vi "FormMain.vi"() -> ()   [LabVIEW 2012]
uses:
  S7Ref.vi
  resultShow.vi
panel:
  out "涂线束色标":bool
  out "请安装线束":bool
  in  "管柱码":string
  in  "countLeft":u32
  out "拾取下轴固定螺丝":bool
  out "安装下轴左转两圈检测":bool=TRUE
  in  "判定设定 2":string[][](table)
  in  "参数设定 2":string[][](table)
  out "takesTime":string
  out "表格控件":string[][](table)
  out "FFT范围 2":string[][](table)
  out "翻起下轴后按左启动按钮下轴平台复位":bool
  out "外泄漏":bool
  out "自由间隙":bool
  out "右转两圈检测":bool
  out "请给总成扫码":bool=TRUE
  out "涂下轴色标":bool
  out "输出扭矩":dbl caption="数值 24" format="%.1f Nm"
  in  "打开按钮":bool
  in  "自动":bool
  out "rigStatus":string="提示信息"
  out "connectionMode":string
  out "productsName":string
  out "userStatus":string
  out "userName":string
  out "双手按启动按钮夹紧工件顶升下轴平台":bool
  out "一号气枪安装下轴":bool=TRUE
  out "双手启动翻转":bool
  out "主观判断是否合格":bool
  out "拆卸下轴后双手启动翻转平位":bool
  out "按右启动键取出工件":bool
  # "下轴总成装配及主观异响鉴别"
  # "广东和氏自动化技术股份有限公司"
  # "GUANGDONG HESH AUTOMATION TECHNOLOGY CO.,LTD."
  # "安装步骤"
  # "完成计数："
  # "："
  # "用时："
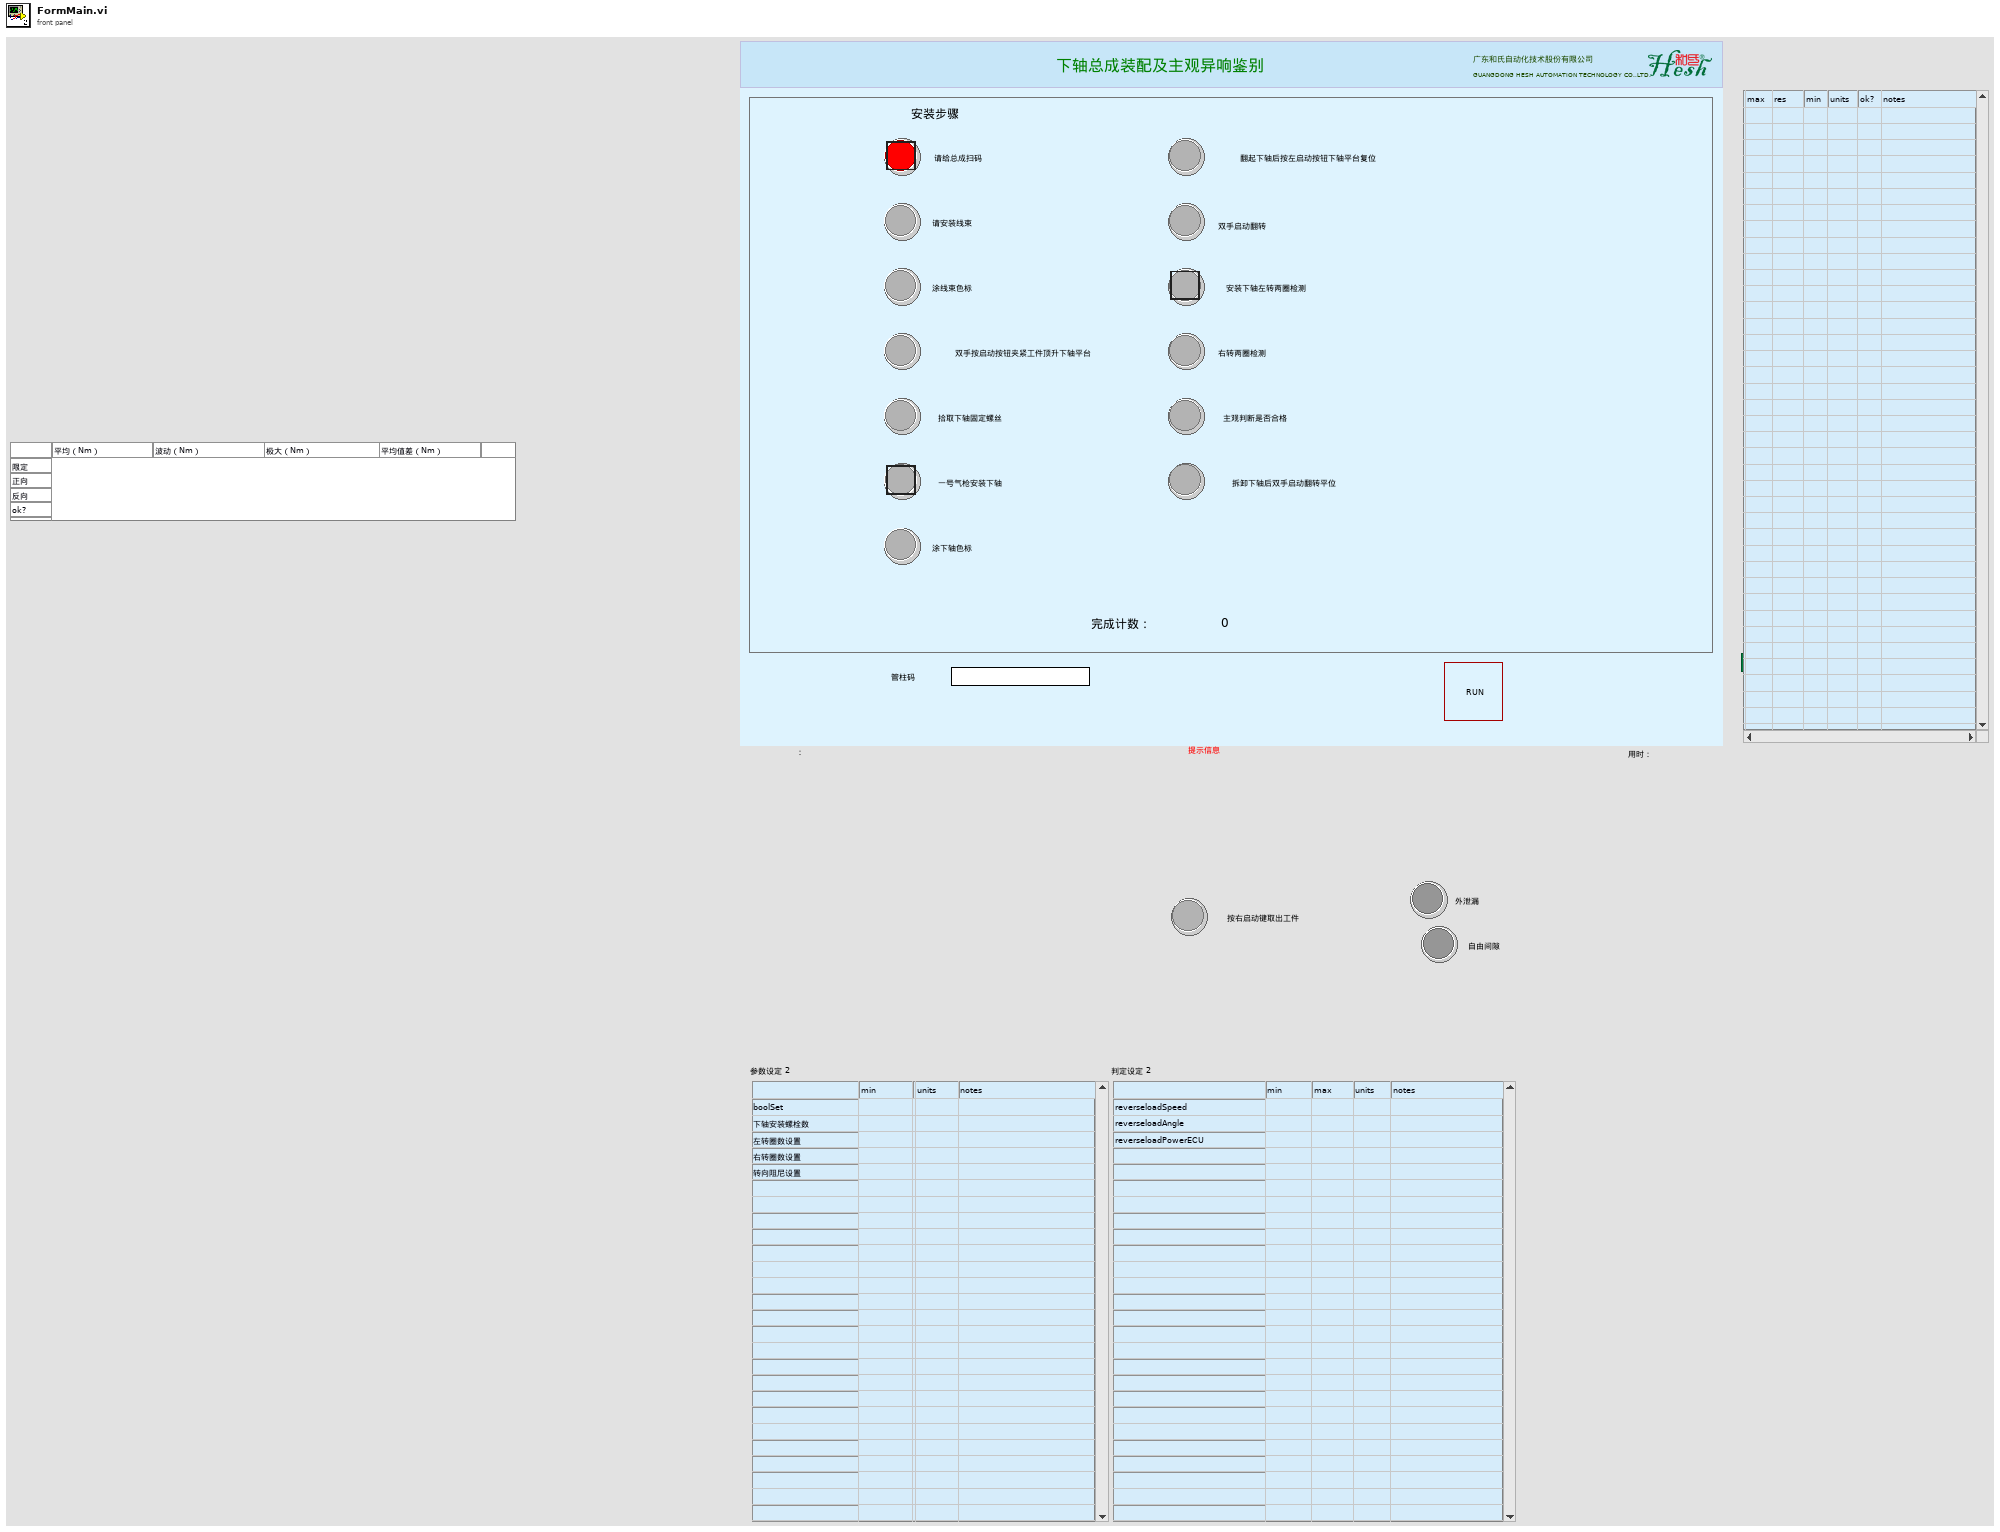
[diagram p1: front panel]
types:
  T1 = enum32{"Invalid", "Standard", "Closed", "Hidden", "Minimized", "Maximized"}
  T2 = cluster{"takesTime":refnum<vi>, "userStatus":refnum<vi>, "userName":refnum<vi>, "connectionMode":refnum<vi>, "productsName":refnum<vi>, "rigStatus":refnum<vi>, "管柱码":refnum<vi>}
  T3 = cluster{"userCode":string, "userName":string, "userStatus":string, "connectionMode":string, "takesTime":string, "countDone":string, "countOK":string, "countNG":string, "rigStatus":string, "productsName":string, "partCode1":string, "partCode2":string, "partCode3":string}
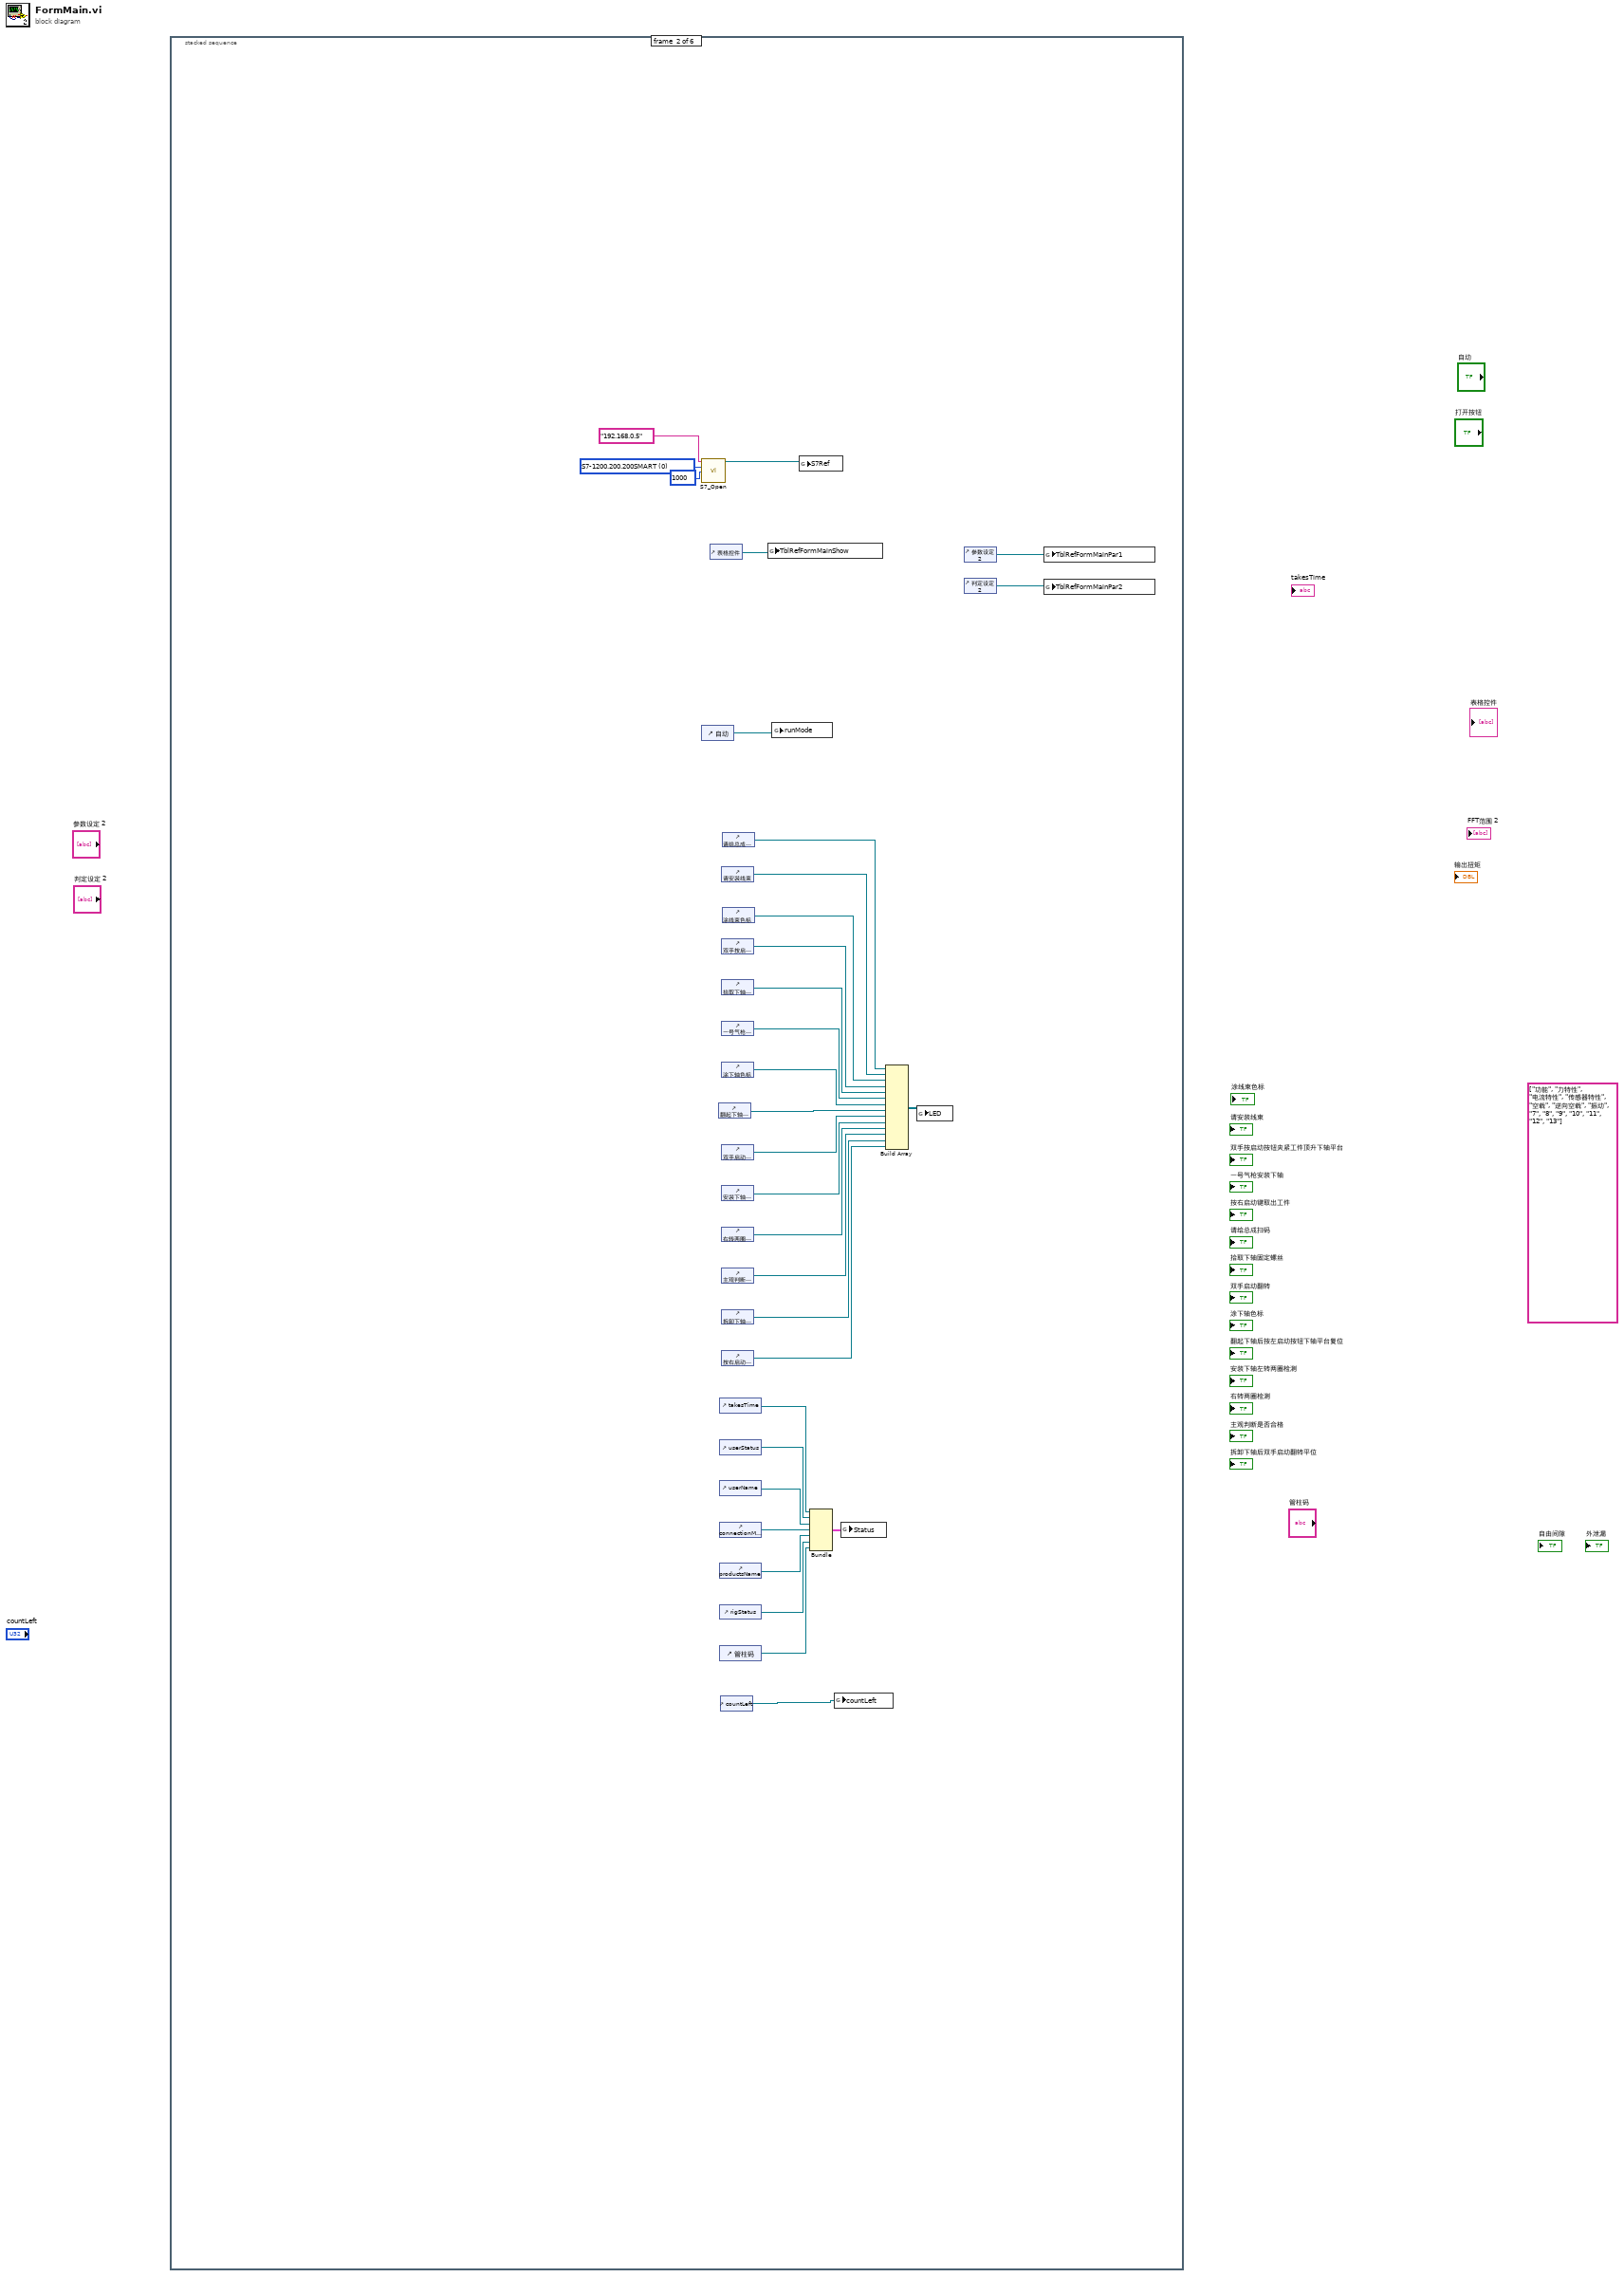
[diagram p0: block diagram]
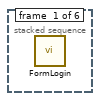
[diagram p2: hidden frame]
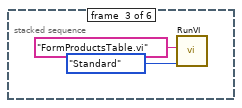
[diagram p3: hidden frame]
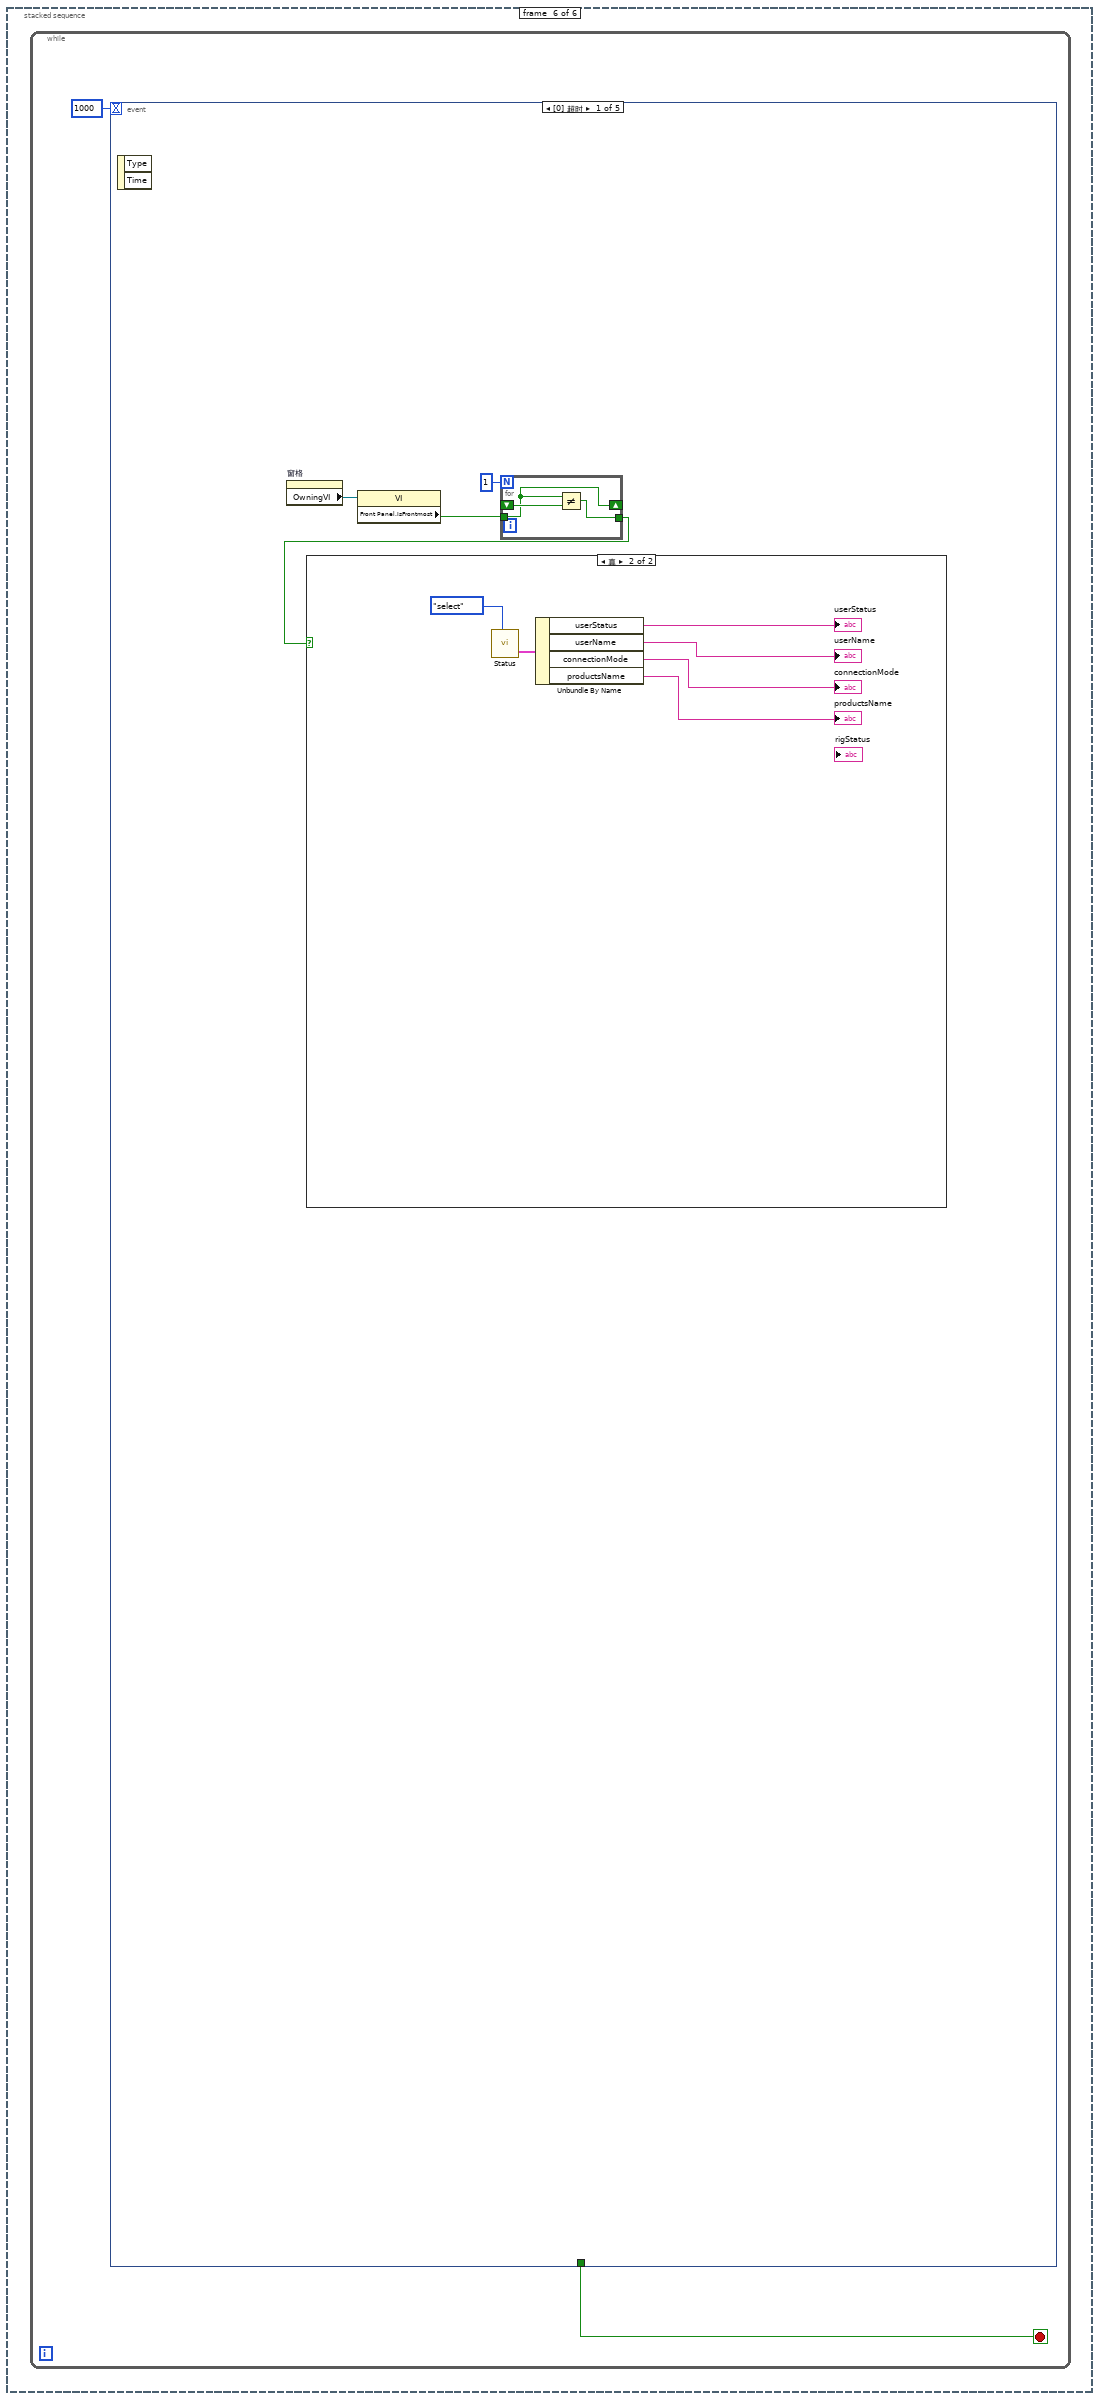
[diagram p6: hidden frame]
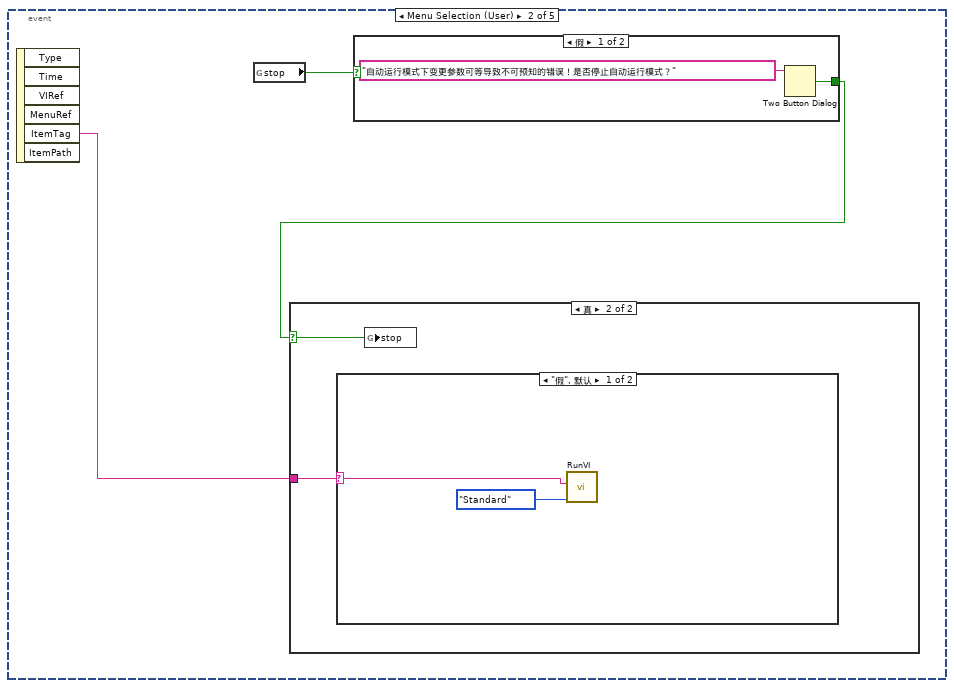
[diagram p8: hidden frame]
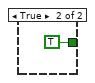
[diagram p9: hidden frame]
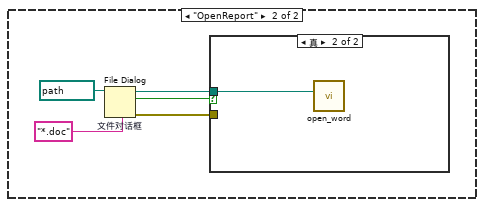
[diagram p11: hidden frame]
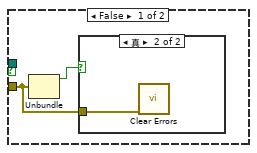
[diagram p12: hidden frame]
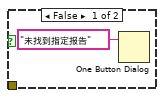
[diagram p13: hidden frame]
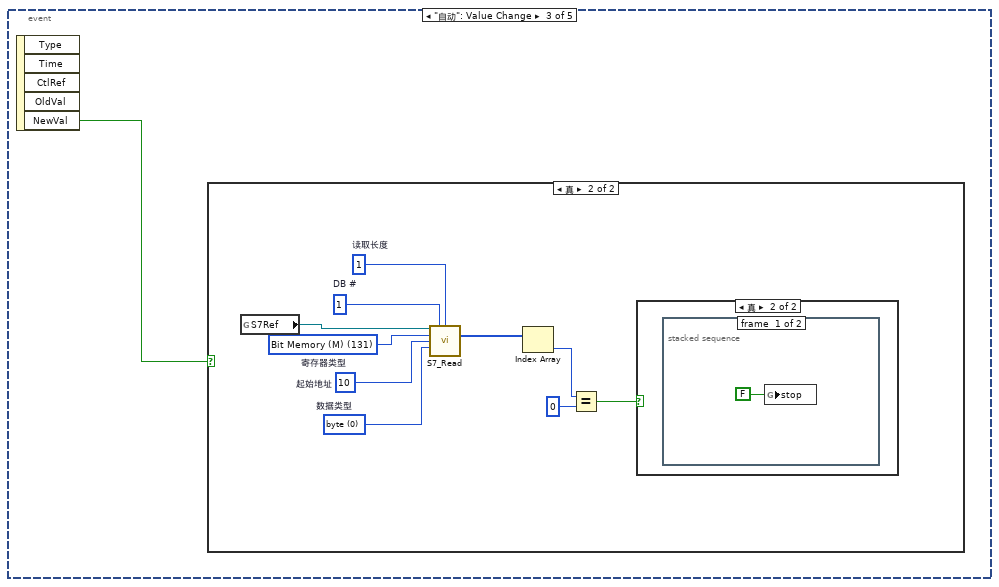
[diagram p14: hidden frame]
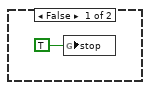
[diagram p15: hidden frame]
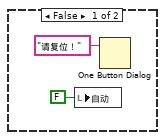
[diagram p16: hidden frame]
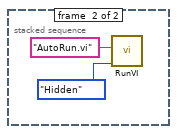
[diagram p17: hidden frame]
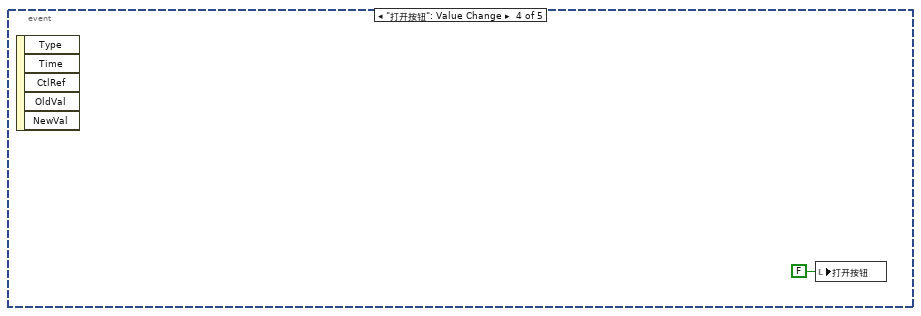
[diagram p18: hidden frame]
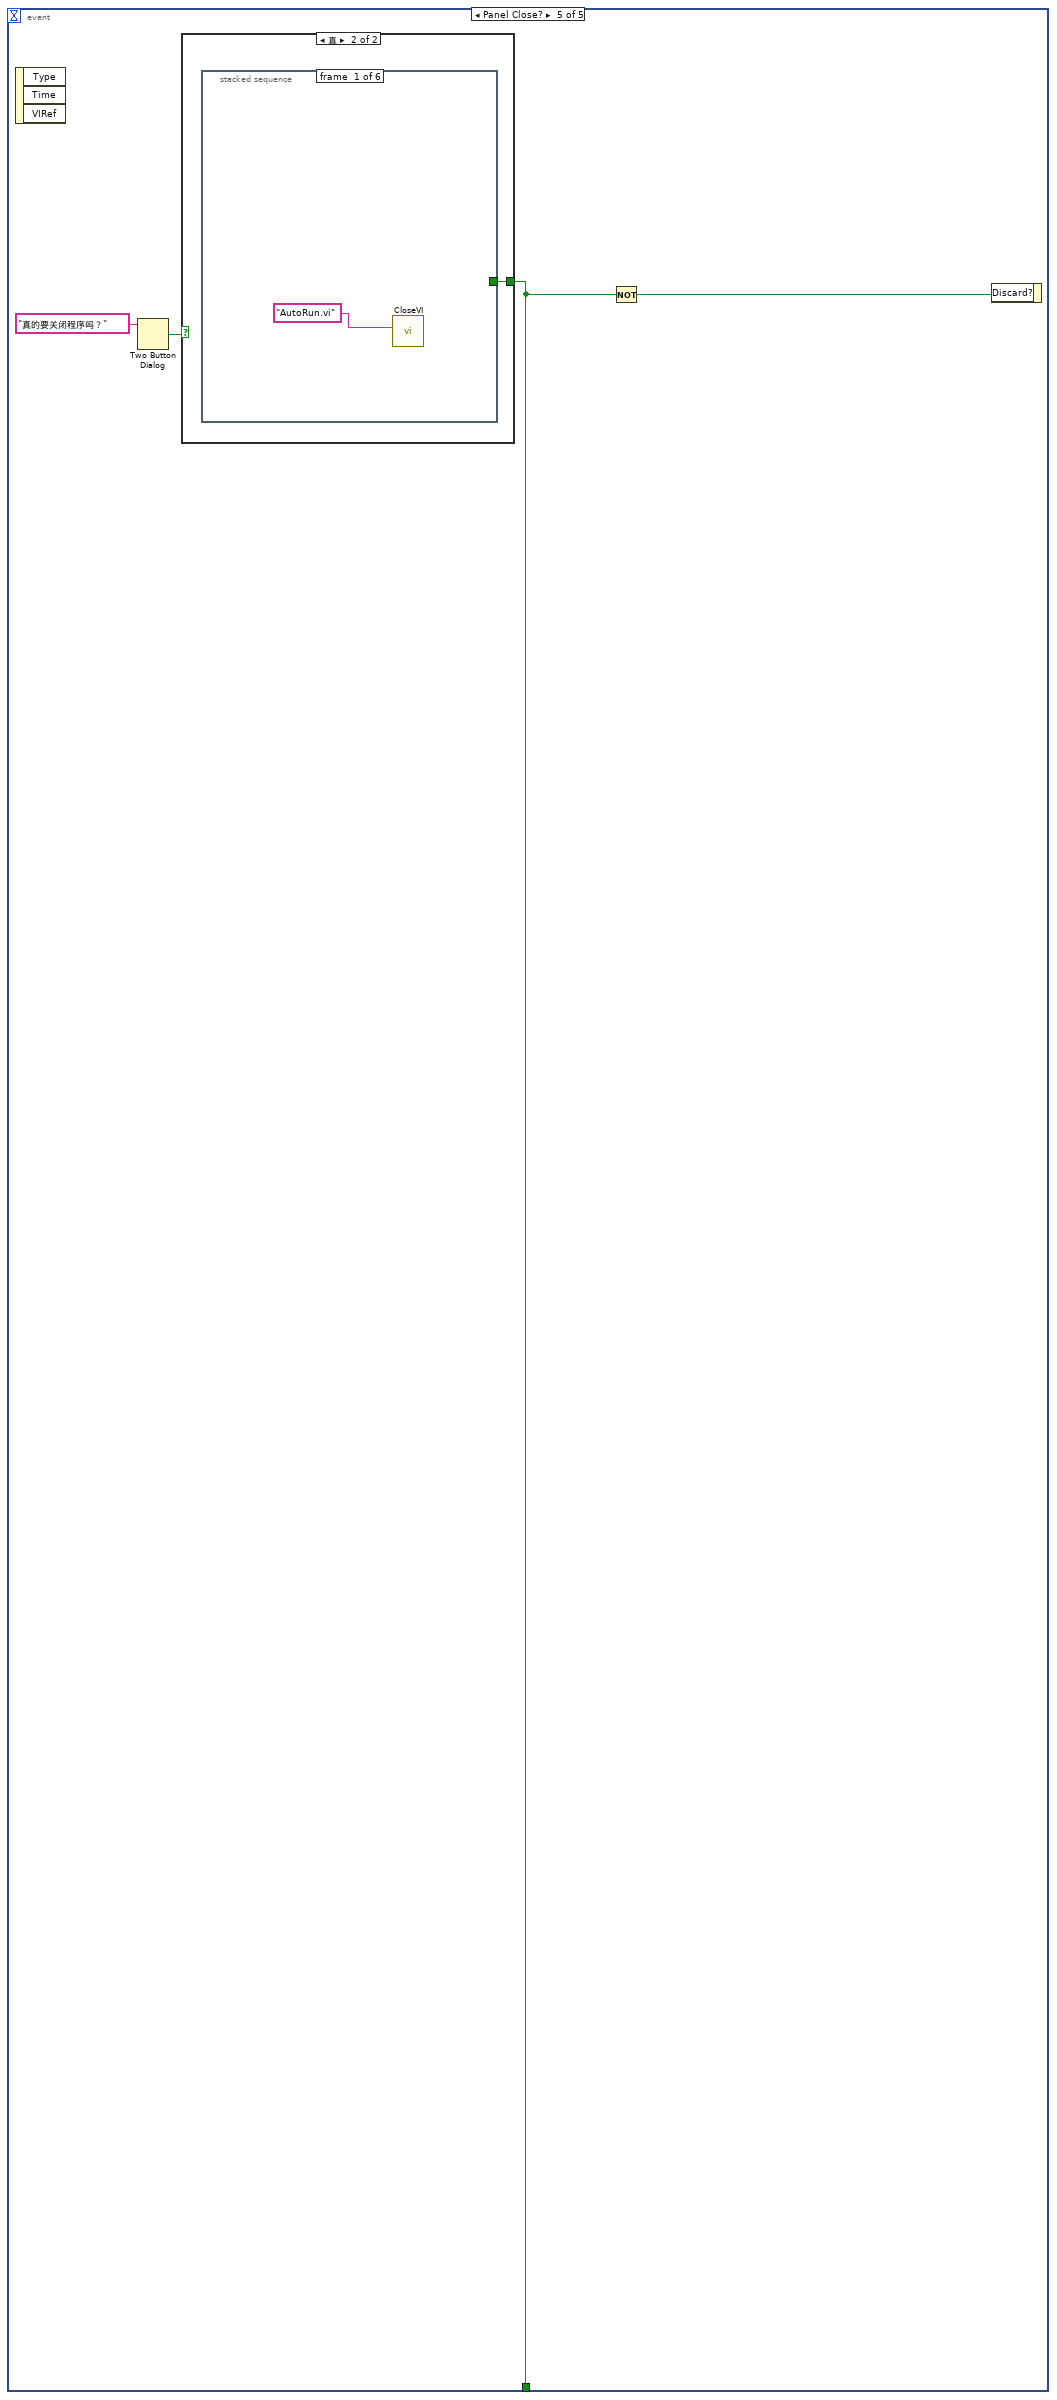
[diagram p19: hidden frame]
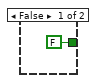
[diagram p20: hidden frame]
diagram:
  (unwired) string[] ["功能", "力特性", "电流特性", "传感器特性", "空载", "逆向空载", "振动", "7", "8", "9", "10", "11", "12", "13"] ("字符串[]")
  n1 = stacked-sequence {
    frame #0 {
      n2 = call "FormLogin.vi"() -> ()  [unwired: 12 in]
    }
    frame #1 {
      w30 = u8 0 items=["S7-1200.200.200SMART"=0, "S7-300"=2, "S7-400"=3] ("PLC 系列")
      n3 = call "S7_Open.vi"("IP 地址"="192.168.0.5", "PLC 系列"=w30, "超时（MS）"=1000) -> ("TCP"=w28:refnum<k5>)  [unwired: 10 in, 2 out]
      n4 = control-ref of="自动"() -> (w27:refnum<vi>)
      n5 = control-ref of="表格控件"() -> (w32:refnum<vi>)
      n6 = control-ref of="翻起下轴后按左启动按钮下轴平台复位"() -> (w4:refnum<vi>)
      n7 = control-ref of="takesTime"() -> (w15:refnum<vi>)
      n8 = control-ref of="userStatus"() -> (w21:refnum<vi>)
      n9 = control-ref of="userName"() -> (w20:refnum<vi>)
      n10 = control-ref of="connectionMode"() -> (w19:refnum<vi>)
      n11 = control-ref of="productsName"() -> (w18:refnum<vi>)
      n12 = control-ref of="rigStatus"() -> (w17:refnum<vi>)
      n13 = control-ref of="管柱码"() -> (w5:refnum<vi>)
      n14 = control-ref of="countLeft"() -> (w12:refnum<vi>)
      n15 = control-ref of="请安装线束"() -> (w2:refnum<vi>)
      n16 = control-ref of="双手按启动按钮夹紧工件顶升下轴平台"() -> (w10:refnum<vi>)
      n17 = control-ref of="拾取下轴固定螺丝"() -> (w8:refnum<vi>)
      n18 = control-ref of="一号气枪安装下轴"() -> (w22:refnum<vi>)
      n19 = control-ref of="涂下轴色标"() -> (w9:refnum<vi>)
      n20 = control-ref of="双手启动翻转"() -> (w23:refnum<vi>)
      n21 = control-ref of="安装下轴左转两圈检测"() -> (w7:refnum<vi>)
      n22 = control-ref of="右转两圈检测"() -> (w6:refnum<vi>)
      n23 = control-ref of="主观判断是否合格"() -> (w24:refnum<vi>)
      n24 = control-ref of="拆卸下轴后双手启动翻转平位"() -> (w25:refnum<vi>)
      n25 = control-ref of="按右启动键取出工件"() -> (w26:refnum<vi>)
      n26 = control-ref of="请给总成扫码"() -> (w3:refnum<vi>)
      n27 = control-ref of="涂线束色标"() -> (w1:refnum<vi>)
      n28 = global write "resultShow.vi" "TblRefFormMainShow"(w32) -> ()
      n29 = global write "resultShow.vi" "runMode"(w27) -> ()
      n30 = global write "S7Ref.vi" "S7Ref"(w28) -> ()
      n31 = Bundle("takesTime"=w15, "userStatus"=w21, "userName"=w20, "connectionMode"=w19, "productsName"=w18, "rigStatus"=w17, "管柱码"=w5) -> (w16:T2)  [unwired: 1 in]
      n32 = global write "resultShow.vi" "countLeft"(w12) -> ()
      n33 = global write "resultShow.vi" "Status"(w16) -> ()
      n34 = Build Array(w3, w2, w1, w10, w8, w22, w9, w4, w23, w7, w6, w24, w25, w26) -> (w11:refnum<vi>[])
      n35 = global write "resultShow.vi" "LED"(w11) -> ()
      n36 = control-ref of="参数设定 2"() -> (w14:refnum<vi>)
      n37 = control-ref of="判定设定 2"() -> (w13:refnum<vi>)
      n38 = global write "resultShow.vi" "TblRefFormMainPar1"(w14) -> ()
      n39 = global write "resultShow.vi" "TblRefFormMainPar2"(w13) -> ()
    }
    frame #2 {
      n40 = call "RunVI.vi"("状态"=T1."Standard", "名称或相对路径"="FormProductsTable.vi") -> ()  [unwired: 9 in, 1 out]
    }
    frame #3 {
    }
    frame #4 {
    }
    frame #5 {
      n41 = while {
        stop <- w36 stop-if-true
        n42 = event shown="[0] 超时" {
          selector: _ -> [_ _ _ _ _]
          dyn-events: _ -> [_ _ _ _ _]
          timeout: 1000 -> [_ _ _ _ _]
          tunnel: [_ _ _ _ w88] -> w36
          event Timeout {
            n43 = event-data() -> ()  [unwired: 1 in, 2 out]
            n44 = property on="窗格" class="Pane"() -> ("OwningVI"=w40:refnum<vi>)  [unwired: 2 in, 2 out]
            n45 = property class="VI"(reference=w40) -> ("Front Panel.IsFrontmost"=w38:bool)  [unwired: 1 in, 2 out]
            n46 = for {
              N: 1 -> [_]
              shift-right: [w48] -> _
              shift-left: _ -> [w49]
              tunnel: w38 -> [w48]
              tunnel: [w47] -> w37
              n47 = Not Equal?(x=w48, y=w49) -> (x != y?=w47:bool)
            }
            n48 = case shown="真" w37 {
              frame False {
              }
              frame True {
                n49 = call "Status.vi"("模式"=enum16{"select", "insert", "update", "delete"}."select") -> ("元素"=w45:T3)  [unwired: 10 in]
                n50 = Unbundle By Name(w45) -> ("userStatus"=→"userStatus":string, "userName"=→"userName":string, "connectionMode"=→"connectionMode":string, "productsName"=→"productsName":string)
              }
            }
          }
          event Menu Selection (User) {
            n51 = event-data() -> ("ItemTag"=w52:string)  [unwired: 1 in, 5 out]
            n52 = global read "全局 3.vi" "stop"() -> (w51:bool)
            n53 = case shown="假" w51 {
              tunnel: [w53 TRUE ("T button?")] -> w50
              frame False {
                n54 = Two Button Dialog(message="自动运行模式下变更参数可等导致不可预知的错误！是否停止自动运行模式？" ("消息")) -> (T button?=w53:bool)  [unwired: 2 in]
              }
              frame True {
              }
            }
            n55 = case shown="真" w50 {
              selector: w50 -> [_ w56]
              tunnel: w52 -> [_ w57]
              frame False {
              }
              frame True {
                n56 = case shown="\"假\", 默认" w57 {
                  selector: w57 -> [w58 _]
                  frame "假", Default {
                    n57 = call "RunVI.vi"("状态"=T1."Standard", "名称或相对路径"=w58) -> ()  [unwired: 9 in, 1 out]
                  }
                  frame "OpenReport" {
                    n58 = File Dialog "文件对话框"(6:"*.doc" ("prompt"), 11:path "D:/报表" ("开始路径")) -> (0:w60:errorcluster, 2:w62:bool, 3:w61:path)  [unwired: 1 in, 5 out]
                    n59 = case shown="真" w62 {
                      tunnel: w61 -> [_ w69]
                      tunnel: w60 -> [w65 _]
                      frame False {
                        n60 = Unbundle(w65) -> ("status"=w66:bool)  [unwired: 2 out]
                        n61 = case shown="真" w66 {
                          tunnel: w65 -> [_ w68]
                          frame False {
                            n62 = One Button Dialog(message="未找到指定报告" ("消息")) -> ()  [unwired: 1 in, 1 out]
                          }
                          frame True {
                            n63 = call <vilib>:"Clear Errors.vi"("error in (no error)"=w68) -> ()  [unwired: 6 in, 1 out]
                          }
                        }
                      }
                      frame True {
                        n64 = call "open_word.vi"("所选路径"=w69) -> ()  [unwired: 11 in]
                      }
                    }
                  }
                }
                n65 = global write "全局 3.vi" "stop"(w56) -> ()
              }
            }
          }
          event "自动": Value Change {
            n66 = event-data() -> ("NewVal"=w70:bool)  [unwired: 1 in, 4 out]
            n67 = case shown="真" w70 {
              frame False {
                n68 = global write "全局 3.vi" "stop"(TRUE ("布尔 1")) -> ()
              }
              frame True {
                w75 = u32 10  # 起始地址
                w77 = u16 0 items=["byte", "word", "Dword"]  # 数据类型
                w78 = u8 131 items=["I/O (P)"=128, "Input (I)"=129, "Output (Q)"=130, "Bit Memory (M)"=131, "Data (DB)"=132, "Instance Data (DI)"=133, "Local Data (L)"=134, "Predecessor Local Data (VL)"=135]  # 寄存器类型
                w79 = u16 1  # 读取长度
                w80 = u16 1  # DB #
                n69 = global read "S7Ref.vi" "S7Ref"() -> (w81:refnum<k5>)
                n70 = call "S7_Read.vi"("TCP"=w81, "DB #"=w80, "读取长度"=w79, "寄存器类型"=w78, "起始地址"=w75, "数据类型"=w77) -> ("数据"=w76:u32[])  [unwired: 6 in, 3 out]
                n71 = Index Array(array=w76) -> (element=w74:u32)  [unwired: 1 in]
                n72 = Equal?(x=w74, y=u32 0) -> (x = y?=w72:bool)
                n73 = case shown="真" w72 {
                  frame False {
                    n74 = local write "自动"(FALSE ("自动")) -> ()
                    n75 = One Button Dialog(message="请复位！" ("消息")) -> ()  [unwired: 1 in, 1 out]
                  }
                  frame True {
                    n76 = stacked-sequence {
                      frame #0 {
                        n77 = global write "全局 3.vi" "stop"(FALSE ("布尔 1")) -> ()
                      }
                      frame #1 {
                        n78 = call "RunVI.vi"("状态"=T1."Hidden", "名称或相对路径"="AutoRun.vi") -> ()  [unwired: 9 in, 1 out]
                      }
                    }
                  }
                }
              }
            }
          }
          event "打开按钮": Value Change {
            n79 = event-data() -> ()  [unwired: 1 in, 5 out]
            n80 = local write "打开按钮"(FALSE ("打开按钮")) -> ()
          }
          event Panel Close? {
            n81 = event-data() -> ()  [unwired: 1 in, 3 out]
            n82 = Two Button Dialog(message="真的要关闭程序吗？" ("消息")) -> (T button?=w89:bool)  [unwired: 2 in]
            n83 = case shown="真" w89 {
              tunnel: [FALSE w93] -> w88
              frame False {
              }
              frame True {
                n84 = stacked-sequence {
                  tunnel: [_ _ _ _ _ w100] -> w93
                  frame #0 {
                    n85 = call "CloseVI.vi"("名称或相对路径"="AutoRun.vi") -> ()  [unwired: 10 in, 1 out]
                  }
                  frame #1 {
                    n86 = shared-variable ".\\共享变量.lvlib\\string_5"("关闭程序中" ("string_5")) -> ()  [unwired: 1 in, 1 out]
                    n87 = global write "全局 3.vi" "stop"(TRUE ("布尔 2")) -> ()
                  }
                  frame #2 {
                    n88 = Wait (ms)(milliseconds to wait=u32 500 ("等待时间（毫秒）")) -> ()  [unwired: 1 out]
                  }
                  frame #3 {
                  }
                  frame #4 {
                    n89 = global read "S7Ref.vi" "S7Ref"() -> (w98:refnum<k5>)
                    n90 = call "S7_Close.vi"("TCP Connection Ref"=w98) -> ()  [unwired: 10 in, 1 out]
                  }
                  frame #5 {
                    w100 = TRUE
                    n91 = case shown="真" TRUE {
                      tunnel: w100 -> [_ w101]
                      frame False {
                      }
                      frame True {
                        n92 = Quit LabVIEW(quit? (T)=w101) -> ()
                      }
                    }
                  }
                }
              }
            }
            n93 = Not(x=w88) -> (.not. x?=w90:bool)
            n94 = event-data("Discard?"=w90) -> ()  [unwired: 1 in, 1 out]
          }
        }
      }
    }
  }
